vi "Check ACNET Device Limits.vi"(8 "error in (no error)":errorcluster, 9 "client handle":T1, 11 "ACNET Devices in":refnum<class "ACNET Devices.lvclass">) -> (0 "error out":errorcluster, 1 "client handle out":T1, 2 "Range Check Results":T2(array[cluster]), 3 "ACNET Devices out":refnum<class "ACNET Devices.lvclass">)   [LabVIEW 2013, in "ACNET Monitor.lvlib"]
uses:
  ACNET Monitor.lvlib
  ACNET Devices.lvclass
  <vilib>/httpClient/ClientHandle.ctl
  ACNET Device.lvclass
  <vilib>/httpClient/LabVIEWHTTPClient.lvlib
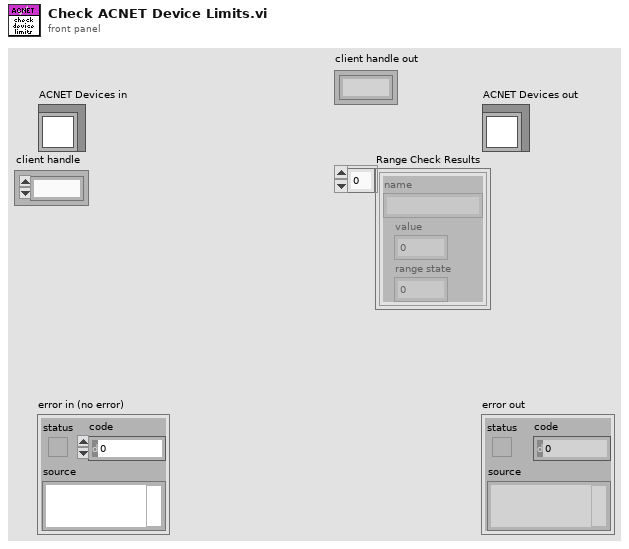
[diagram p1: front panel]
types:
  T1 = typedef "LabVIEWHTTPClient.lvlib/ClientHandle.ctl" = refnum<k1>
  T2 = cluster{"name":string, "value":dbl, "range state":i8}[]
  T3 = cluster{"name":string, "value":dbl, "range state":i8}
  T4 = cluster{"Name":string, "Units":string, "Value":string}[]
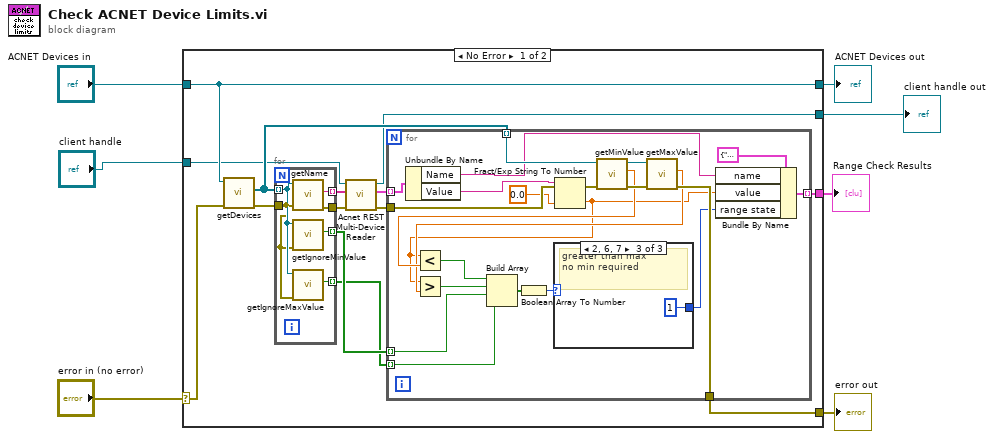
[diagram p0: block diagram]
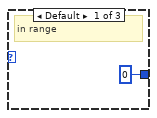
[diagram p2: hidden frame]
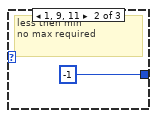
[diagram p3: hidden frame]
diagram:
  n1 = case shown="No Error" "error in (no error)" {
    selector: "error in (no error)" -> [w17 w54]
    tunnel: [w19 w54] -> w6
    tunnel: [w18 w53] -> w4
    tunnel: "ACNET Devices in" -> [w18 w53]
    tunnel: [w14 _] -> w3
    tunnel: "client handle" -> [w11 w52]
    tunnel: [w10 w52] -> w1
    frame No Error {
      n2 = call-dynamic "getDevices.vi"("error in (no error)"=w17, "ACNET Devices in"=w18) -> ("error out"=w15:errorcluster, "Devices"=w16:refnum<class "ACNET Device.lvclass">[])  [unwired: 7 in, 1 out]
      n3 = for {
        tunnel: w16 -> [w49] mode=indexing
        tunnel: w15 -> [w48]
        tunnel: [w51] -> w13 mode=indexing
        tunnel: [w50] -> w21
        tunnel: [w47] -> w9 mode=indexing
        tunnel: [w46] -> w8 mode=indexing
        n4 = call-dynamic "getName.vi"("error in (no error)"=w48, "ACNET Device in"=w49) -> ("error out"=w50:errorcluster, "name"=w51:string)  [unwired: 7 in, 1 out]
        n5 = call-dynamic "getIgnoreMinValue.vi"("error in (no error)"=w48, "ACNET Device in"=w49) -> ("ignoreMinValue"=w47:bool)  [unwired: 7 in, 2 out]
        n6 = call-dynamic "getIgnoreMaxValue.vi"("error in (no error)"=w48, "ACNET Device in"=w49) -> ("ignoreMaxValue"=w46:bool)  [unwired: 7 in, 2 out]
      }
      n7 = call "Acnet REST Multi-Device Reader.vi"("error in (no error)"=w21, "Devices"=w13, "client handle"=w11) -> ("error out"=w20:errorcluster, "ACNET Device Readings"=w12:T4, "client handle out"=w10:T1)  [unwired: 6 in]
      n8 = for {
        tunnel: w12 -> [w37] mode=indexing
        tunnel: w16 -> [w42] mode=indexing
        tunnel: w20 -> [w39]
        tunnel: [w38] -> w19
        tunnel: [w31] -> w14 mode=indexing
        tunnel: w9 -> [w24] mode=indexing
        tunnel: w8 -> [w23] mode=indexing
        n9 = Unbundle By Name(w37) -> ("Name"=w32:string, "Value"=w33:string)
        n10 = Fract/Exp String To Number(string=w33, default (0 dbl)=0.0 ("default (0 I32)")) -> (number=w22:dbl)  [unwired: 2 in, 1 out]
        n11 = call-dynamic "getMinValue.vi"("error in (no error)"=w39, "ACNET Devices in"=w42) -> ("error out"=w41:errorcluster, "minValue"=w26:dbl, "ACNET Devices out"=w40:refnum<class "ACNET Device.lvclass">)  [unwired: 7 in]
        n12 = Less?(x=w22, y=w26) -> (x < y?=w30:bool)
        n13 = call-dynamic "getMaxValue.vi"("error in (no error)"=w41, "ACNET Devices in"=w40) -> ("error out"=w38:errorcluster, "maxValue"=w25:dbl)  [unwired: 7 in, 1 out]
        n14 = Greater?(x=w22, y=w25) -> (0:w29:bool)
        n15 = Build Array(w30, w29, w24, w23) -> (w27:bool[])
        n16 = Boolean Array To Number(Boolean array=w27) -> (number=w28:u32)
        n17 = case shown="2, 6, 7" w28 {
          tunnel: [0 -1 1] -> w35
          frame Default {
            # "in range"
          }
          frame 1, 9, 11 {
            # "less then min\nno max required"
          }
          frame 2, 6, 7 {
            # "greater than max\nno min required"
          }
        }
        n18 = Bundle By Name(cluster=T3 {"name"="", "value"=0.0, "range state"=0}, "name"=w32, "value"=w22, "range state"=w35) -> (w31:T3)
      }
    }
    frame Error {
    }
  }
  "error out" <- w6
  "ACNET Devices out" <- w4
  "Range Check Results" <- w3
  "client handle out" <- w1
